vi "Step 2 - Perform Notch Filtering (Notch).vi"() -> ()   [LabVIEW 2023]
doc: "Demonstrates how to use the DFD Filtering VI to perform filtering.\n\nComplete the following steps to use this VI.\n1) Run the VI.\n2) Observe the Signals graph to find the effect of notch filtering. Use the graph tools to zoom in the graph to understand the converging process of the infinite impulse response (IIR) notch filtering.\n3) Examine the block diagram for information about using the DFD Filtering VI."
uses:
  <vilib>/addons/Digital Filter Design/Design.llb/DFD IIR Notch Peak Design by Q.vi
  <vilib>/addons/Digital Filter Design/Process.llb/DFD Filtering (Wfm).vi
  <vilib>/addons/Digital Filter Design/NI_DigFilterLicensed.lvlib
  <vilib>/measure/NI_MAPro.lvlib
panel:
  out "Signals":waveform(dbl)[](graph)=[{"t0"=timestamp(0 s since 1904-01-01), "dt"=1.0, "Y"=[]}, {"t0"=timestamp(0 s since 1904-01-01), "dt"=1.0, "Y"=[]}]
  # "Select Help>>Show Context Help and move the cursor over the VI icon for more information."
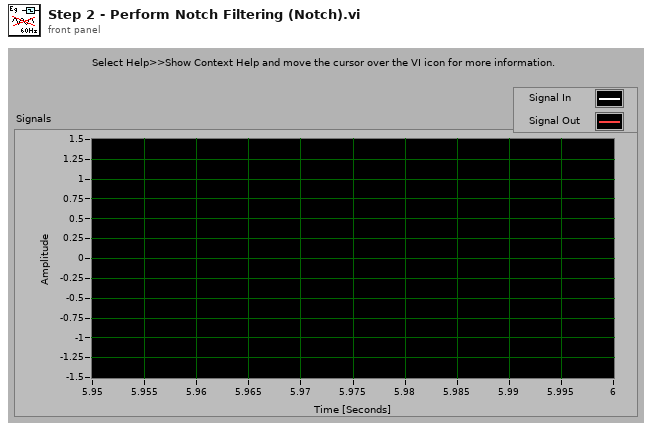
[diagram p1: front panel]
types:
  T1 = typedef "NI_DigFilterLicensed.lvlib/DFD Filter Obj.ctl" = cluster{"mSRate_Fs":dbl, "mSRate_Version":string, "mSRate_Comments":string, "mSRate_OrgCoef":T2, "mSRate_CurCoef":T2, "mSRate_Quantized?":bool, "mSRate_QCoef":T2, "mSRate_QSettings":T4[], "mSRate_Order":i32, "mSRate_Scaling":cluster{"mSRate_ScaleByPowerOf2?":bool, "mSRate_ScaleType":T6}}
  T2 = typedef "NI_DigFilterLicensed.lvlib/DFD Filter Coef.ctl" = cluster{"type":T3, "gain":dbl, "coef a (k)":dbl[], "coef b (v)":dbl[]}
  T3 = typedef "NI_DigFilterLicensed.lvlib/DFD Filter Structure Type Selector.ctl" = enum16{"Undefined", "FIR Direct Form", "FIR Direct Form Transposed", "FIR Symmetric", "FIR Antisymmetric", "IIR Direct Form I", "IIR Direct Form I Transposed", "IIR Direct Form II", "IIR Direct Form II Transposed", "IIR Cascaded Second Order Sections Form I", "IIR Cascaded Second Order Sections Form I Transposed", "IIR Cascaded Second Order Sections Form II", "IIR Cascaded Second Order Sections Form II Transposed", "Lattice Allpass (basic sections)", "Lattice Allpass (one multiplier sections)", "Lattice Allpass (normalized sections)", "Lattice AR (basic sections)", "Lattice AR (one multiplier sections)", "Lattice AR (normalized sections)", "Lattice MA (minimum phase)", "Lattice MA (maximum phase)", "Lattice ARMA (basic sections)", "Lattice ARMA (one multiplier sections)", "Lattice ARMA (normalized sections)"}
  T4 = typedef "NI_DigFilterLicensed.lvlib/dfd_Internal Quantization Settings.ctl" = cluster{"source":T5, "wl":i16, "iwl":i16, "overflow mode":enum16{"Saturation", "Wrap"}, "rounding mode":enum16{"Nearest", "Truncation"}, "signed?":bool}
  T5 = typedef "NI_DigFilterLicensed.lvlib/dfd_Internal Quantization Srcs.ctl" = u16
  T6 = typedef "NI_DigFilterLicensed.lvlib/DFD Coef Norm Type.ctl" = enum16{"No Norm", "Time Domain 1-Norm", "Time Domain 2-Norm", "Time Domain Inf-Norm"}
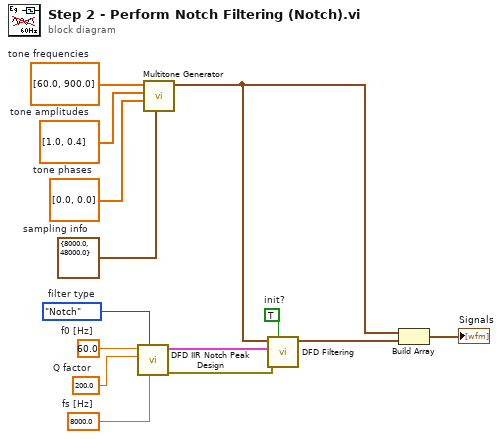
[diagram p0: block diagram]
diagram:
  w3 = dbl[] [0.0, 0.0]  # tone phases
  w5 = dbl[] [60.0, 900.0]  # tone frequencies
  w4 = dbl[] [1.0, 0.4]  # tone amplitudes
  w6 = cluster{"Fs":dbl, "#s":dbl} {"Fs"=8000.0, "#s"=48000.0}  # sampling info
  w9 = TRUE  # init?
  w11 = 8000.0  # fs [Hz]
  w12 = 200.0  # Q factor
  w13 = 60.0  # f0 [Hz]
  w14 = enum16{"Notch", "Peak"}."Notch"  # filter type
  n1 = call-poly <vilib>:"DFD IIR Notch Peak Design.vi"("fs [Hz]"=w11, "filter type"=w14, "Q factor"=w12, "f0 [Hz]"=w13) -> ("error out"=w1:errorcluster, "filter out"=w10:T1)  [unwired: 1 in, 5 out]
  n2 = call <vilib>:"Multitone Generator.vi"("sampling info"=w6, "tone phases"=w3, "tone amplitudes"=w4, "tone frequencies"=w5) -> ("signal out"=w2:waveform(dbl))  [unwired: 4 in, 3 out]
  n3 = call-poly <vilib>:"DFD Filtering.vi"("init? (F)"=w9, "error in (no error)"=w1, "filter"=w10, "signal in"=w2) -> ("signal out"=w8:waveform(dbl))  [unwired: 7 out]
  n4 = Build Array(w2, w8) -> (→"Signals":waveform(dbl)[])
